vi "Test_LogValueEvent_LogClass_MatchInterfaceMethodCallFormattoString.vi"(8 "error in (no error)":errorcluster, 11 "TestCase in":refnum<class "TestLogValue.lvclass">) -> (0 "error out":errorcluster, 3 "TestCase out":refnum<class "TestLogValue.lvclass">)   [LabVIEW 2019, in "TestLogValue.lvclass"]
uses:
  TestLogValue.lvclass
  Source/Composed Log/Types/Log Level.ctl
  Source/Composed Log/LoggerReference/LoggerReference.lvclass/LoggerReference.ctl
  Source/LVQueue Sink/LVQueue Sink.lvclass/LVQueue Sink.ctl
  272d61b2-f49c-486c-9daf-337ffb054b40.vi
  154dbc8a-62f5-4aa1-ad82-2a3c469f95b7.vi
  Source/Composed Log/LoggerReference/Return Aggregate Queues.vi
  Source/Composed Log/LoggerReference/Add Aggregate Log.vi
  272d61b2-f49c-486c-9daf-337ffb054b40.vi/e3ab99c8-d28f-4cf0-a218-d4cd80a9e25e.vi
  154dbc8a-62f5-4aa1-ad82-2a3c469f95b7.vi/df1f5a9e-bfaa-4a04-adf5-95c46504be52.vi
  Source/Composed Log/LoggerReference/Get Valid Event Time.vi
  Source/Composed Log/LoggerReference/Log Event.vi
  Source/Composed Log/LoggerReference/Send Add Sink.vi
  Source/Composed Log/LoggerReference/Log.vi
  Source/Composed Log/LoggerReference/Remove Stale Logs.vi
  Source/LVQueue Sink/LVQueue Sink.lvclass
  C:/CS/Log/Source/Composed Log/Log Sink/Log Sink.lvclass
  Source/Composed Log/Application Logger/Launch Worker Loop.vi
  Source/Composed Log/LoggerReference/Initialize Logger Instance.vi
  Source/Composed Log/LoggerReference/LoggerReference.lvclass
  Source/Composed Log/IErrorFormat/IErrorFormat.lvclass
  Source/Composed Log/Log Sink/Log Sink.lvclass
  <vilib>/addons/_JKI Toolkits/VI Tester/TestCase.llb/TestCase.lvclass
  Source/Composed Log/Composed Log.lvlib
  C:/Program Files (x86)/National Instruments/LabVIEW 2019/vi.lib/addons/_JKI Toolkits/VI Tester/TestCase.llb/TestCase.lvclass
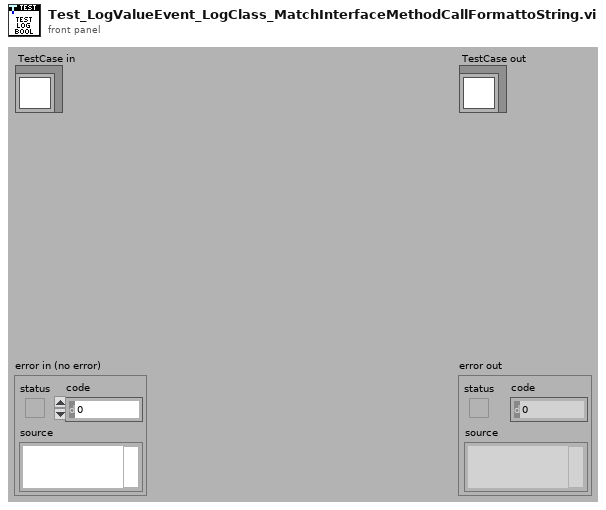
[diagram p1: front panel]
types:
  T1 = typedef "Composed Log.lvlib/Log Level.ctl" = enum16{"Debug", "Info", "Warning", "Error", "Critical"}
  T2 = typedef "Composed Log.lvlib/Log Packet.ctl" = cluster{"Data To Log":string, "Source":string, "Event Level":T1, "Event Time":timestamp}
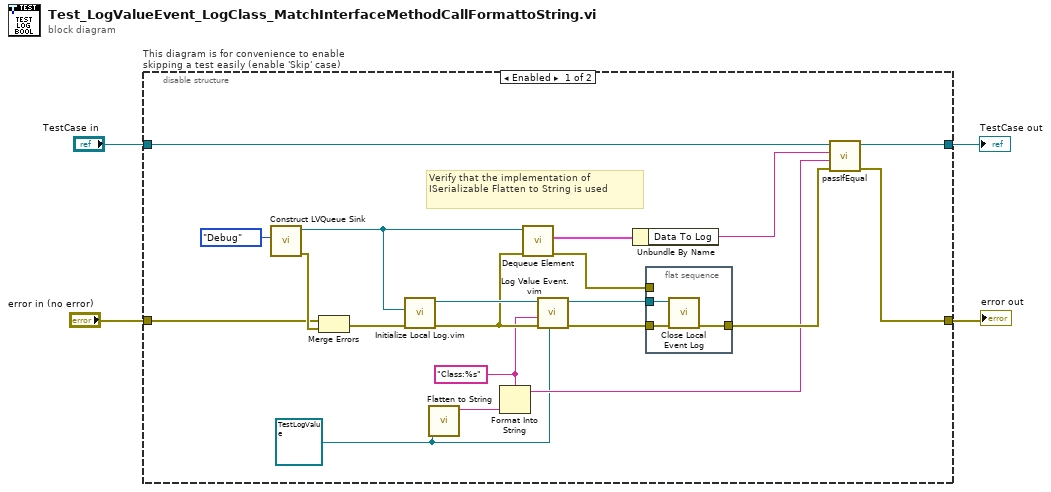
[diagram p0: block diagram]
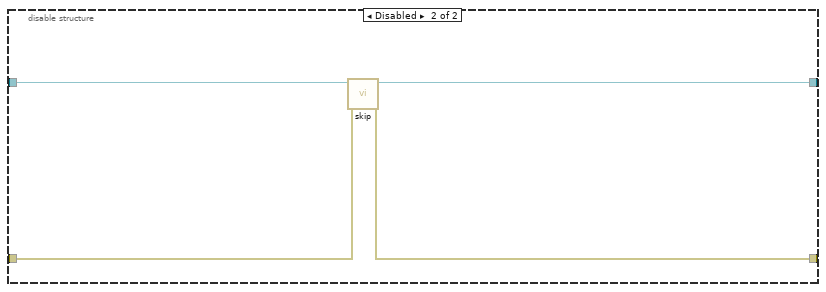
[diagram p2: hidden frame]
diagram:
  n1 = disable-structure "This diagram is for convenience to enable skipping a test easily (enable 'Skip' case)" shown="Enabled" {
    disable-tunnel: "TestCase in" -> [w18 w31]
    disable-tunnel: [w17 w29] -> w1
    disable-tunnel: [w15 w30] -> w3
    disable-tunnel: "error in (no error)" -> [w16 w28]
    frame Enabled {
      w6 = refnum<class "TestLogValue.lvclass"> refnum ("TestLogValue.lvclass")
      w10 = "Class:%s" ("Data To Log")
      # "Verify that the implementation of ISerializable Flatten to String is used"
      n2 = call "Construct LVQueue Sink.vi"("LogLevel"=Log_Level."Debug") -> ("error out"=w21:errorcluster, "LVQueue Sink out"=w19:refnum<class "LVQueue Sink.lvclass">)  [unwired: 9 in]
      n3 = Merge Errors(w16, w21) -> (w20:errorcluster)
      n4 = call "Initialize Local Log.vim"("error in (no error)"=w20, "Startup Sink(s)"=w19) -> ("error out"=w13:errorcluster, "Log Instance Reference"=w14:refnum<class "LoggerReference.lvclass">)  [unwired: 7 in, 1 out]
      n5 = call-dynamic "Flatten to String.vi"("TestLogValue in"=w6) -> ("Flattened Class"=w5:string)  [unwired: 9 in, 1 out]
      n6 = Format Into String(format string=w10, w5) -> (resulting string=w8:string)  [unwired: 2 in, 1 out]
      n7 = call "Dequeue Element.vi"("error in (no error)"=w13, "LVQueue Sink in"=w19) -> ("error out"=w24:errorcluster, "Log Packet"=w22:T2)  [unwired: 6 in, 2 out]
      n8 = call "Log Value Event.vim"("Value(s)"=w6, "error in (no error)"=w13, "Log Message Format String"=w10, "LoggerReference in"=w14) -> ("error out"=w12:errorcluster, "LoggerReference out"=w11:refnum<class "LoggerReference.lvclass">)  [unwired: 6 in]
      n9 = Unbundle By Name(w22) -> ("Data To Log"=w9:string)
      n10 = flat-sequence {
        tunnel: [w26] -> w23
        tunnel: w12 -> [w27]
        tunnel: w24 -> [_]
        tunnel: w11 -> [w25]
        frame #0 {
          n11 = call "Close Local Event Log.vi"("error in (no error)"=w27, "Log Instance"=w25) -> ("error out"=w26:errorcluster)  [unwired: 9 in]
        }
      }
      n12 = call-dynamic "passIfEqual.vi"("error in (no error)"=w23, "y"=w8, "x"=w9, "TestCase in"=w18) -> ("error out"=w15:errorcluster, "TestCase out"=w17:refnum<class "TestLogValue.lvclass">)  [unwired: 6 in]
    }
    frame Disabled {
      # "skip test result while test is under development"
      n13 = call <vilib>:"skip.vi"("error in (no error)"=w28, "TestCase in"=w31) -> ("error out"=w30:errorcluster, "TestCase out"=w29:refnum<class "TestLogValue.lvclass">)  [unwired: 8 in]
    }
  }
  "error out" <- w3
  "TestCase out" <- w1
